vi "Enqueue Message (Array).vi"(6 "优先消息？数组":bool[](array[boolean]), 8 "error in (no error)":cluster{"状态":bool, "代码":i32, "源":string} caption="错误输入（无错误）", 9 "消息数据数组":variant[](array[variant]), 10 "消息数组":string[](array[string]), 11 "消息队列":refnum<queue>) -> (0 "error out":cluster{"状态":bool, "代码":i32, "源":string} caption="错误输出", 3 "消息队列副本":refnum<queue>)   [LabVIEW 2014, in "Message Queue.lvlib"]
doc: "对于标准消息，将消息加入队列。对于优先消息，将消息加入队列的头部。"
uses:
  Message Queue.lvlib
  Message Cluster.ctl
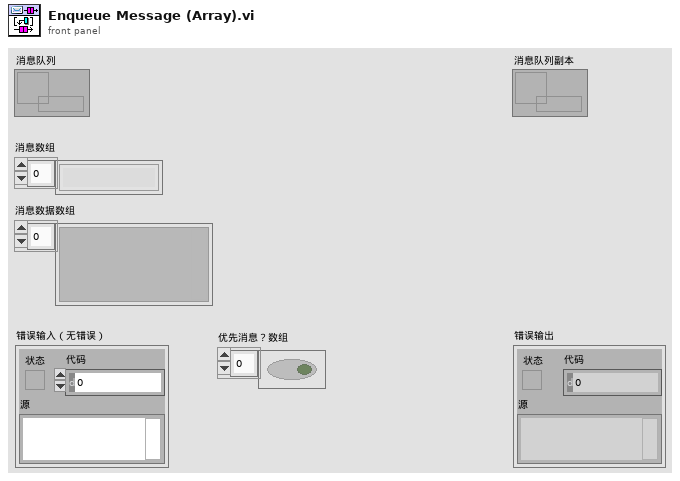
[diagram p1: front panel]
types:
  T1 = typedef "Message Queue.lvlib/Message Cluster.ctl" = cluster{"消息":string, "消息数据":variant}
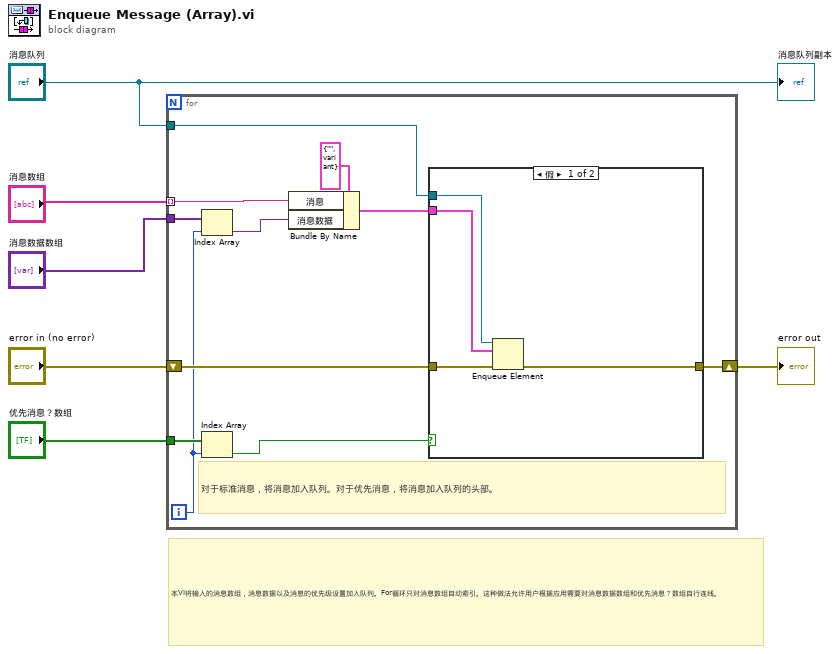
[diagram p0: block diagram]
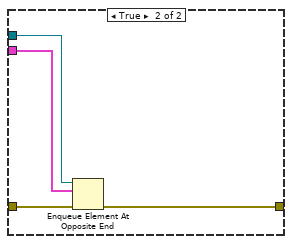
[diagram p2: hidden frame]
diagram:
  # "本VI将输入的消息数组，消息数据以及消息的优先级设置加入队列。For循环只对消息数组自动索引。这种做法允许用户根据应用需要对消息数据数组和优先消息？数组自行连线。"
  n1 = for {
    tunnel: "消息数组" -> [w16] mode=indexing
    tunnel: "消息数据数组" -> [w11]
    tunnel: "优先消息？数组" -> [w9]
    tunnel: "消息队列" -> [w13]
    shift-right: [w14] -> w2
    shift-left: "error in (no error)" -> [w15]
    i -> [w7]
    # "对于标准消息，将消息加入队列。对于优先消息，将消息加入队列的头部。"
    n2 = Index Array(array=w11, index=w7) -> (element=w10:variant)
    n3 = Index Array(array=w9, index=w7) -> (element=w8:bool)
    n4 = Bundle By Name(cluster=T1 {"消息"="", "消息数据"=variant} ("Message Cluster"), "消息"=w16, "消息数据"=w10) -> (w12:T1)
    n5 = case shown="假" w8 {
      tunnel: w15 -> [w21 w25]
      tunnel: [w20 w24] -> w14
      tunnel: w13 -> [w19 w23]
      tunnel: w12 -> [w18 w22]
      frame False {
        n6 = Enqueue Element(queue=w19, element=w18, error in (no error)=w21) -> (error out=w20:errorcluster)  [unwired: 1 in, 2 out]
      }
      frame True {
        n7 = Enqueue Element At Opposite End(queue=w23, element=w22, error in (no error)=w25) -> (error out=w24:errorcluster)  [unwired: 1 in, 2 out]
      }
    }
  }
  "error out" <- w2
  "消息队列副本" <- "消息队列"
